vi "Get Item Property.vi"(8 "error in (no error)":errorcluster, 9 "Default Value":variant, 10 "Property Name":string, 11 "Item Reference in":T1 format="%.0x") -> (0 "error out":errorcluster, 1 "Value":variant, 3 "Item Reference out":T1 format="%.0x", 4 "found":bool)   [LabVIEW 2013, in "Hierarchy Framework.lvlib" / "Item.lvclass"]
doc: "Returns the <B>Value</B> of a specific item <B>Property Name</B>. Properties do not inherit within a custom device, so <B>Item Ref in</B> must reference the specific item on which the property is set. \n\nFor instances with a <B>Default Value</B> input, the <B>Value</B> output returns this value if the <B>Property Name</B> is not found for the specified item. Wire data to the <B>Default Value</B> input to determine the polymorphic instance to use or manually select the instance."
uses:
  Item.lvclass
  Ctls/Item Reference.ctl
  Generic/Generic.lvclass
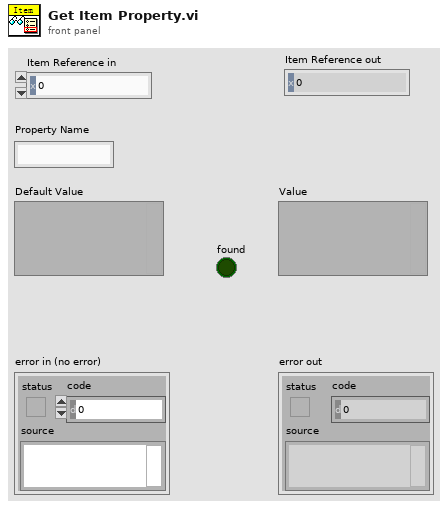
[diagram p1: front panel]
types:
  T1 = typedef "Hierarchy Framework.lvlib/Item.lvclass/Item Reference.ctl" = u64
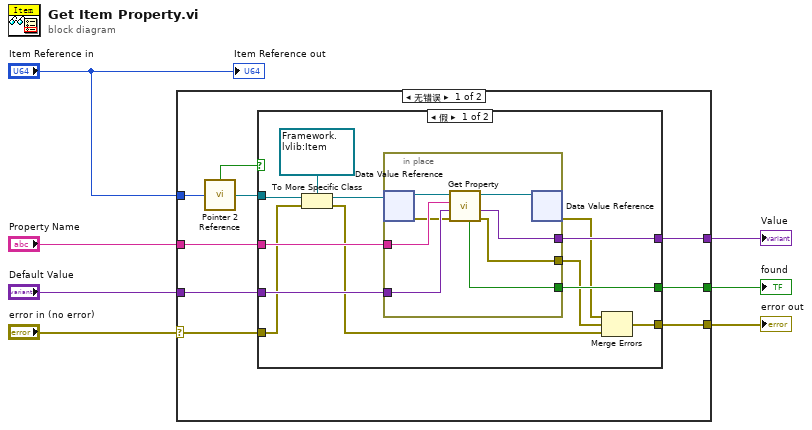
[diagram p0: block diagram]
diagram:
  n1 = case shown="无错误" "error in (no error)" {
    selector: "error in (no error)" -> [w11 w40]
    tunnel: "Item Reference in" -> [w10 _]
    tunnel: "Property Name" -> [w16 _]
    tunnel: "Default Value" -> [w15 w39]
    tunnel: [w14 _] -> w4
    tunnel: [w13 w39] -> w3
    tunnel: [w12 w40] -> w2
    frame No Error {
      n2 = call "Pointer 2 Reference.vi"("Pointer"=w10) -> ("Not A Refnum?"=w9:bool, "Generic Reference"=w8:refnum<data-value>)
      n3 = case shown="假" w9 {
        tunnel: w16 -> [w28 _]
        tunnel: w15 -> [w27 w38]
        tunnel: [w26 _] -> w14
        tunnel: [w25 w38] -> w13
        tunnel: w11 -> [w20 w37]
        tunnel: [w23 w37] -> w12
        tunnel: w8 -> [w21 _]
        frame False {
          n4 = To More Specific Class(target class=refnum<data-value> refnum ("Item"), reference=w21, error in=w20) -> (specific class reference=w18:refnum<data-value>, error out=w19:errorcluster)
          n5 = in-place {
            in-place-border: w28 -> [w35]
            in-place-border: w27 -> [w34]
            in-place-border: [w30] -> w26
            in-place-border: [w31] -> w25
            in-place-border: [w29] -> w22
            n6 = in-place-dvr #1(w18) -> (w36:refnum<class "Item.lvclass">, w33:errorcluster)
            n7 = call-dynamic "Get Property.vi"("error in (no error)"=w33, "Default Value"=w34, "Property Name"=w35, "Item输入"=w36) -> ("error out"=w29:errorcluster, "Value"=w31:variant, "Item输出"=w32:refnum<class "Item.lvclass">, "found"=w30:bool)  [unwired: 4 in]
            n8 = in-place-dvr #1(w32) -> (w24:errorcluster)  [unwired: 1 out]
          }
          n9 = Merge Errors(w24, w22, w19) -> (w23:errorcluster)
        }
        frame True {
        }
      }
    }
    frame Error {
    }
  }
  "found" <- w4
  "Value" <- w3
  "error out" <- w2
  "Item Reference out" <- "Item Reference in"
